vi "Escape String.vi"(1 "Remove Escapes? (False)":bool, 2 "Escapes":cluster{"String":string, "Escape":string}[](array[cluster]), 3 "String in":string) -> (0 "String out":string)   [LabVIEW 2020]
doc: "Adds or Removes escapes to or from a string.\n\n<B>String in</B> - The string to handle escapes in,\n<B>Escapes</B> - The escape patterns to handle. When adding escapes, they are added in the order of the array. If removing escapes, they are removed in reverse order.\n<B>Remove Escapes?</B> - Should the escapes be added or removed.\n<B>String out</B> - The resulting string with the escapes handled."
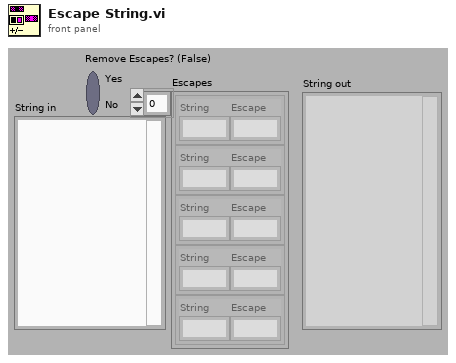
[diagram p1: front panel]
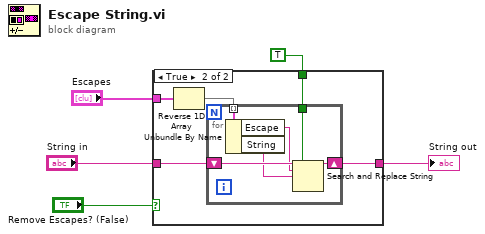
[diagram p0: block diagram]
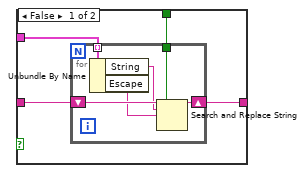
[diagram p2: hidden frame]
diagram:
  n1 = case shown="True" "Remove Escapes? (False)" {
    tunnel: "Escapes" -> [w8 w19]
    tunnel: "String in" -> [w9 w20]
    tunnel: TRUE ("replace all? (F)") -> [w7 w18]
    tunnel: [w6 w17] -> w1
    frame False {
      n2 = for {
        shift-right: [w13] -> w6
        shift-left: w9 -> [w15]
        tunnel: w8 -> [w12] mode=indexing
        tunnel: w7 -> [w14]
        n3 = Unbundle By Name(w12) -> ("String"=w11:string, "Escape"=w10:string)
        n4 = Search and Replace String(replace all?=w14, input string=w15, search string=w11, replace string=w10) -> (result string=w13:string)  [unwired: 4 in, 3 out]
      }
    }
    frame True {
      n5 = Reverse 1D Array(array=w19) -> (reversed array=w16:cluster{"String":string, "Escape":string}[])
      n6 = for {
        shift-right: [w24] -> w17
        shift-left: w20 -> [w26]
        tunnel: w16 -> [w23] mode=indexing
        tunnel: w18 -> [w25]
        n7 = Unbundle By Name(w23) -> ("Escape"=w22:string, "String"=w21:string)
        n8 = Search and Replace String(replace all?=w25, input string=w26, search string=w22, replace string=w21) -> (result string=w24:string)  [unwired: 4 in, 3 out]
      }
    }
  }
  "String out" <- w1
